vi "Read Count.vi"(8 "error in (no error)":errorcluster, 11 "StandardFunction in":refnum<class "StandardFunction.lvclass">) -> (0 "error out":errorcluster, 2 "Count":u16, 3 "StandardFunction out":refnum<class "StandardFunction.lvclass">)   [LabVIEW 2014]
uses:
  StandardFunction.lvclass
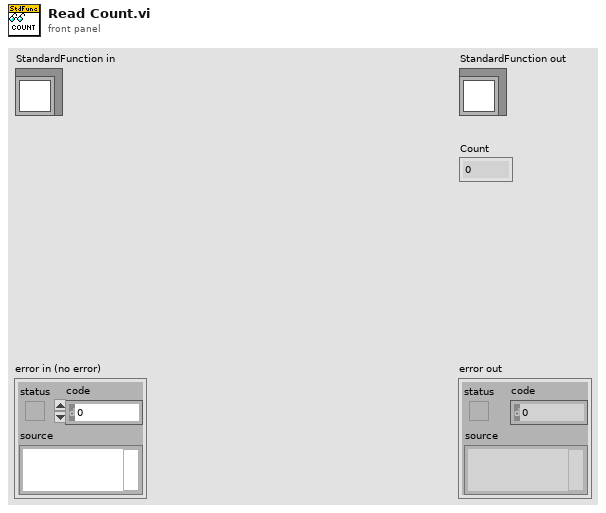
[diagram p1: front panel]
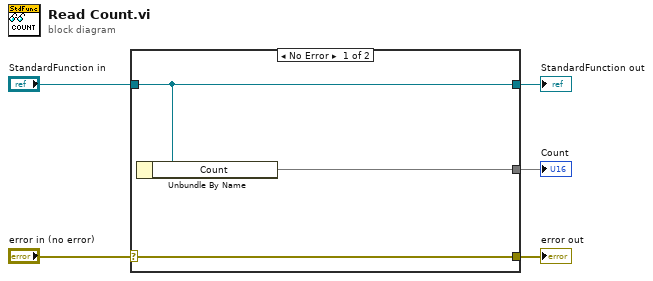
[diagram p0: block diagram]
diagram:
  n1 = case shown="No Error" "error in (no error)" {
    selector: "error in (no error)" -> [w8 w9]
    tunnel: [w8 w9] -> w4
    tunnel: [w7 w10] -> w2
    tunnel: "StandardFunction in" -> [w7 w10]
    tunnel: [w6 _] -> w1
    frame No Error {
      n2 = Unbundle By Name(w7) -> ("Count"=w6)
    }
    frame Error {
    }
  }
  "error out" <- w4
  "StandardFunction out" <- w2
  "Count" <- w1
